vi "FinalizeHWI.vi"(8 "error in (no error)":errorcluster, 10 "Master Device in":refnum<class "Master Device.lvclass">, 11 "NI Card in":refnum<class "NI Card.lvclass">) -> (0 "error out":errorcluster, 2 "Master Device out":refnum<class "Master Device.lvclass">, 3 "NI Card out":refnum<class "NI Card.lvclass">)   [LabVIEW 2013, in "NI Card.lvclass"]
uses:
  NI Card.lvclass
  Master Device/Master Device.lvclass
  NI Card.lvclass/NI Card.ctl
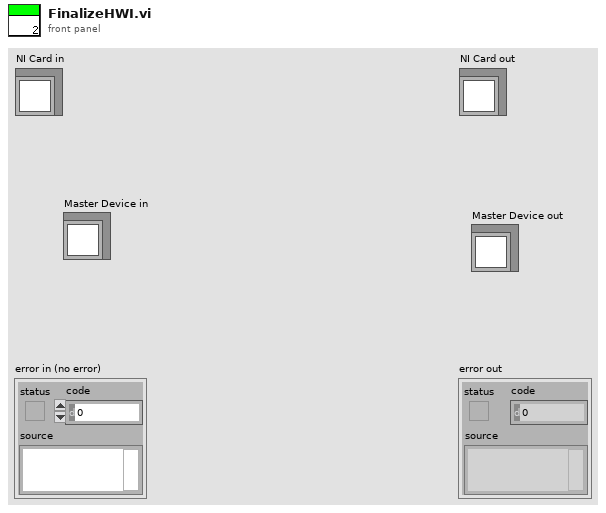
[diagram p1: front panel]
types:
  T1 = typedef "RampInfo.ctl" = cluster{"Table Ramp Index":i32, "Ramp Time":dbl, "Number of Steps":i32, "VLIW Array Index":i32}
  T2 = cluster{"Triggering":bool[][], "Ramp Info":T1[], "VLIW Array":cluster{"Output Bits":u32, "Data Field":u32, "OP Code":u8, "Delay Count":u64}[]}
  T3 = cluster{"Parsed analog ramp":dbl[][], "Parsed Digital Data":bool[][]}[]
  T4 = cluster{"Parsed analog ramp":dbl[][], "Parsed Digital Data":bool[][]}
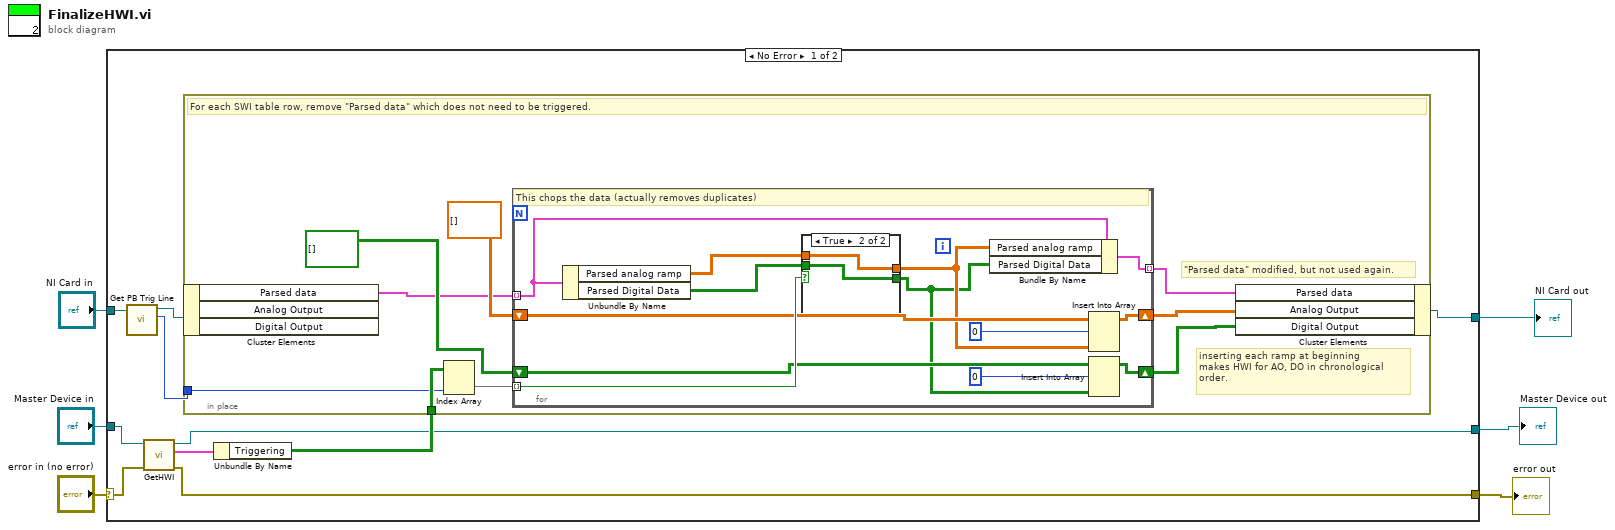
[diagram p0: block diagram]
diagram:
  n1 = case shown="No Error" "error in (no error)" {
    selector: "error in (no error)" -> [w13 w43]
    tunnel: [w7 w43] -> w5
    tunnel: [w8 w42] -> w4
    tunnel: "NI Card in" -> [w12 w42]
    tunnel: "Master Device in" -> [w11 w41]
    tunnel: [w9 w41] -> w1
    frame No Error {
      n2 = call-dynamic "Get PB Trig Line.vi"("Device in"=w12) -> ("PB Trigger Line"=w14:u16, "Device out"=w10:refnum<class "NI Card.lvclass">)  [unwired: 8 in, 1 out]
      n3 = call-dynamic "GetHWI.vi"("error in (no error)"=w13, "Master Device in"=w11) -> ("error out"=w7:errorcluster, "Hardware Image"=w16:T2, "Master Device out"=w9:refnum<class "Master Device.lvclass">)  [unwired: 7 in]
      n4 = Unbundle By Name(w16) -> ("Triggering"=w15:bool[][])
      n5 = in-place {
        in-place-border: w15 -> [w25]
        in-place-border: w14 -> [w24]
        # "\"Parsed data\" modified, but not used again."
        # "inserting each ramp at beginning\nmakes HWI for AO, DO in chronological\norder."
        # "For each SWI table row, remove \"Parsed data\" which does not need to be triggered."
        n6 = in-place-cluster #1(w10) -> ("Parsed data"=w19:T3)  [unwired: 2 out]
        n7 = Index Array(array=w25, index (col)=w24) -> (element=w23:bool[])  [unwired: 1 in]
        n8 = for {
          tunnel: w19 -> [w29] mode=indexing
          tunnel: w23 -> [w38] mode=indexing
          tunnel: [w26] -> w22 mode=indexing
          shift-right: [w37] -> w18
          shift-left: dbl[][] [] ("Parsed Analog Data") -> [w35]
          shift-right: [w36] -> w17
          shift-left: bool[][] [] ("Parsed Digital Data") -> [w34]
          # "This chops the data (actually removes duplicates)"
          n9 = Unbundle By Name(w29) -> ("Parsed analog ramp"=w31:dbl[][], "Parsed Digital Data"=w30:bool[][])
          n10 = case shown="True" w38 {
            tunnel: [_ w40] -> w28
            tunnel: w31 -> [_ w40]
            tunnel: w30 -> [_ w39]
            tunnel: [_ w39] -> w27
            frame False {
            }
            frame True {
            }
          }
          n11 = Bundle By Name(cluster=w29, "Parsed analog ramp"=w28, "Parsed Digital Data"=w27) -> (w26:T4)
          n12 = Insert Into Array(array=w35, index (row)=0, new element=w28) -> (w37:dbl[][])  [unwired: 1 in]
          n13 = Insert Into Array(array=w34, index (row)=0, new element=w27) -> (w36:bool[][])  [unwired: 1 in]
        }
        n14 = in-place-cluster #1("Parsed data"=w22, "Analog Output"=w18, "Digital Output"=w17) -> (w8:refnum<class "NI Card.lvclass">)
      }
    }
    frame Error {
    }
  }
  "error out" <- w5
  "NI Card out" <- w4
  "Master Device out" <- w1
